vi "WriteBitData.vi"(3 "ErrorIn":errorcluster, 4 "ByteArray":u8[](array[numeric])=[64, 50, 185, 216, 109, 115, 113, 40, 12, 0, 0, 254, 0, 1, 2, 3, 4, 5, 3, 6, 0, 0, 0, 0, 82, 111, 98, 101, 114, 116, 13, 10], 5 "Write FilePath":path=path "/Freundlein/Users/Bobby/Documents/Bobbys Stuff/Research/ASP/Code/Labview/WVD-MCSupdate/tempShare/NewMCSDataWriter/WriterTesting.bin") -> (0 "ErrorOut":errorcluster)   [LabVIEW 2012]
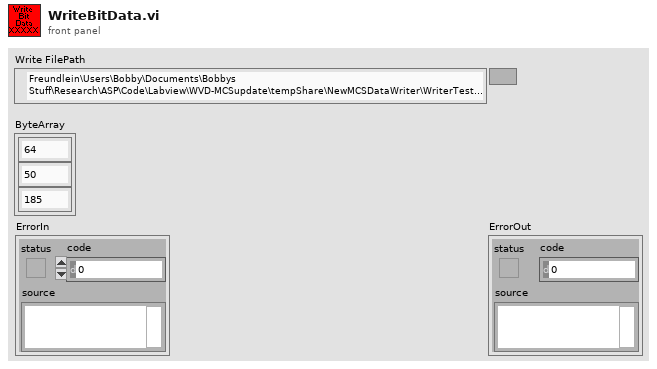
[diagram p1: front panel]
types:
  T1 = enum16{"open", "replace", "create", "open or create", "replace or create", "replace or create with confirmation"}
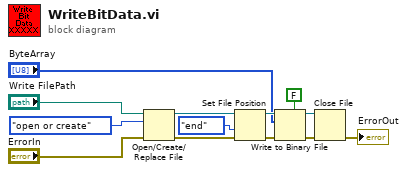
[diagram p0: block diagram]
diagram:
  n1 = Open/Create/Replace File(file path (use dialog)="Write FilePath", error in="ErrorIn", operation (0:open)=T1."open or create") -> (refnum out=w11:refnum<file>, error out=w9:errorcluster)  [unwired: 3 in, 1 out]
  n2 = Set File Position(refnum=w11, from (0:start)=enum16{"start", "end", "current"}."end", error in=w9) -> (refnum out=w7:refnum<file>, error out=w6:errorcluster)  [unwired: 1 in]
  n3 = Write to Binary File(file (use dialog)=w7, data="ByteArray", error in=w6, 5:FALSE ("prepend array or string size? (T)")) -> (refnum out=w2:refnum<file>, error out=w3:errorcluster)  [unwired: 2 in, 1 out]
  n4 = Close File(refnum=w2, error in=w3) -> (error out=→"ErrorOut":errorcluster)  [unwired: 1 out]
